vi "Initialize.vi"(8 "DD_通道名称列表":string[](array[string]), 9 "通道信息":T1[](array[typedef]), 10 "采样率":i32, 11 "原始采样率":i32) -> (3 "通知器输出":refnum<notifier>)   [LabVIEW 2018, in "DataDisplay.lvlib"]
uses:
  DataDisplay.lvlib
  TypeDefine/DD_ChannelInfo.ctl
  TypeDefine/DD_DataStream.ctl
  DD_Parameter.vi
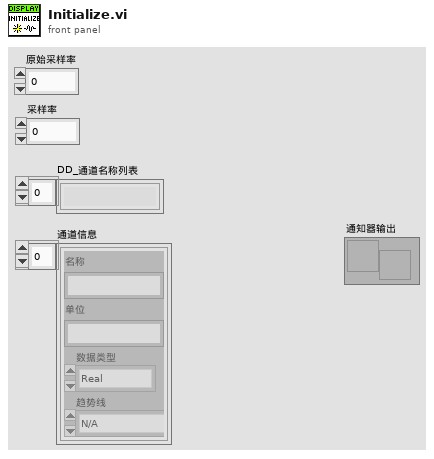
[diagram p1: front panel]
types:
  T1 = typedef "DataDisplay.lvlib/DD_ChannelInfo.ctl" = cluster{"名称":string, "单位":string, "数据类型":enum16{"Real", "Int"}, "趋势线":enum16{"N/A", "X", "Y"}}
  T2 = typedef "DataDisplay.lvlib/DD_DataStream.ctl" = cluster{"Data":dbl[]}[]
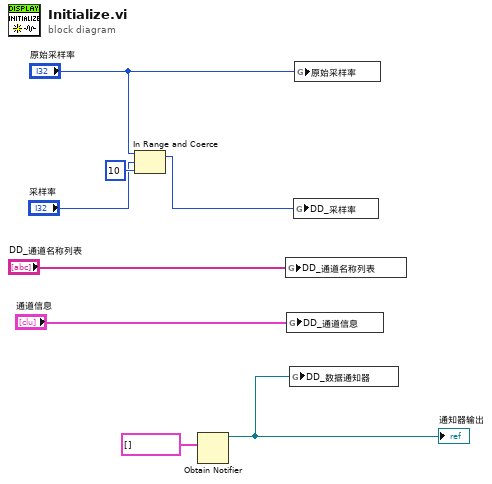
[diagram p0: block diagram]
diagram:
  n1 = In Range and Coerce(upper limit="原始采样率", x="采样率", lower limit=10 ("下限")) -> (coerced(x)=w1:i32)  [unwired: 1 out]
  n2 = Obtain Notifier(notification data type=T2 [] ("Data")) -> (notifier out=w6:refnum<notifier>)  [unwired: 3 in, 2 out]
  "通知器输出" <- w6
  n3 = global write "DD_Parameter.vi" "DD_通道名称列表"("DD_通道名称列表") -> ()
  n4 = global write "DD_Parameter.vi" "DD_通道信息"("通道信息") -> ()
  n5 = global write "DD_Parameter.vi" "DD_数据通知器"(w6) -> ()
  n6 = global write "DD_Parameter.vi" "DD_采样率"(w1) -> ()
  n7 = global write "DD_Parameter.vi" "原始采样率"("原始采样率") -> ()
